vi "Schedule Global.vi"() -> ()   [LabVIEW 2023]
uses:
  Schedule.ctl
panel:
  in  "Multicolumn Listbox":T1
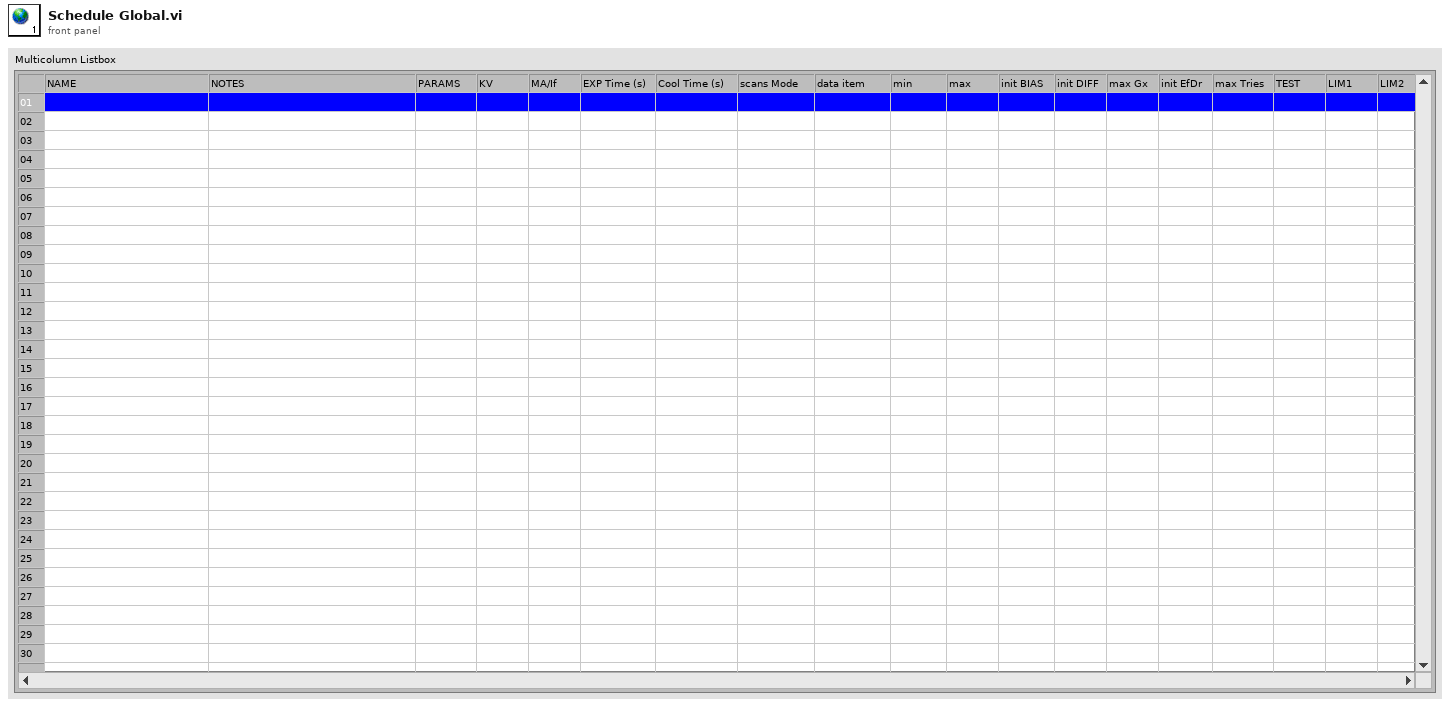
[diagram p1: front panel]
types:
  T1 = typedef "Schedule.ctl" = i32
diagram:
